vi "Shut down.vi"(8 "Error In":errorcluster, 11 "GUI":T1) -> ()   [LabVIEW 2011]
uses:
  Controls/Top Level Control.ctl
  <vilib>/NI/AMC/Message Queue.ctl
  <vilib>/NI/AMC/Message.ctl
  <vilib>/NI/Tools/Keyed Array/KeyedArray.ctl
  Controls/ListBox Test Record.ctl
  Controls/DVR of CSV Tests Data.ctl
  Controls/CSVs Tests Data.ctl
  Controls/Test Column Data.ctl
  Controls/Options DVR.ctl
  Controls/Options.ctl
  <userlib>/_MGI/Application Control/MGI Save & Restore Settings/MGI SRS Command Enum.ctl
  <vilib>/NI/AMC/AMC.lvlib
  <vilib>/NI/Tools/Keyed Array/Tools_KeyedArray.lvlib
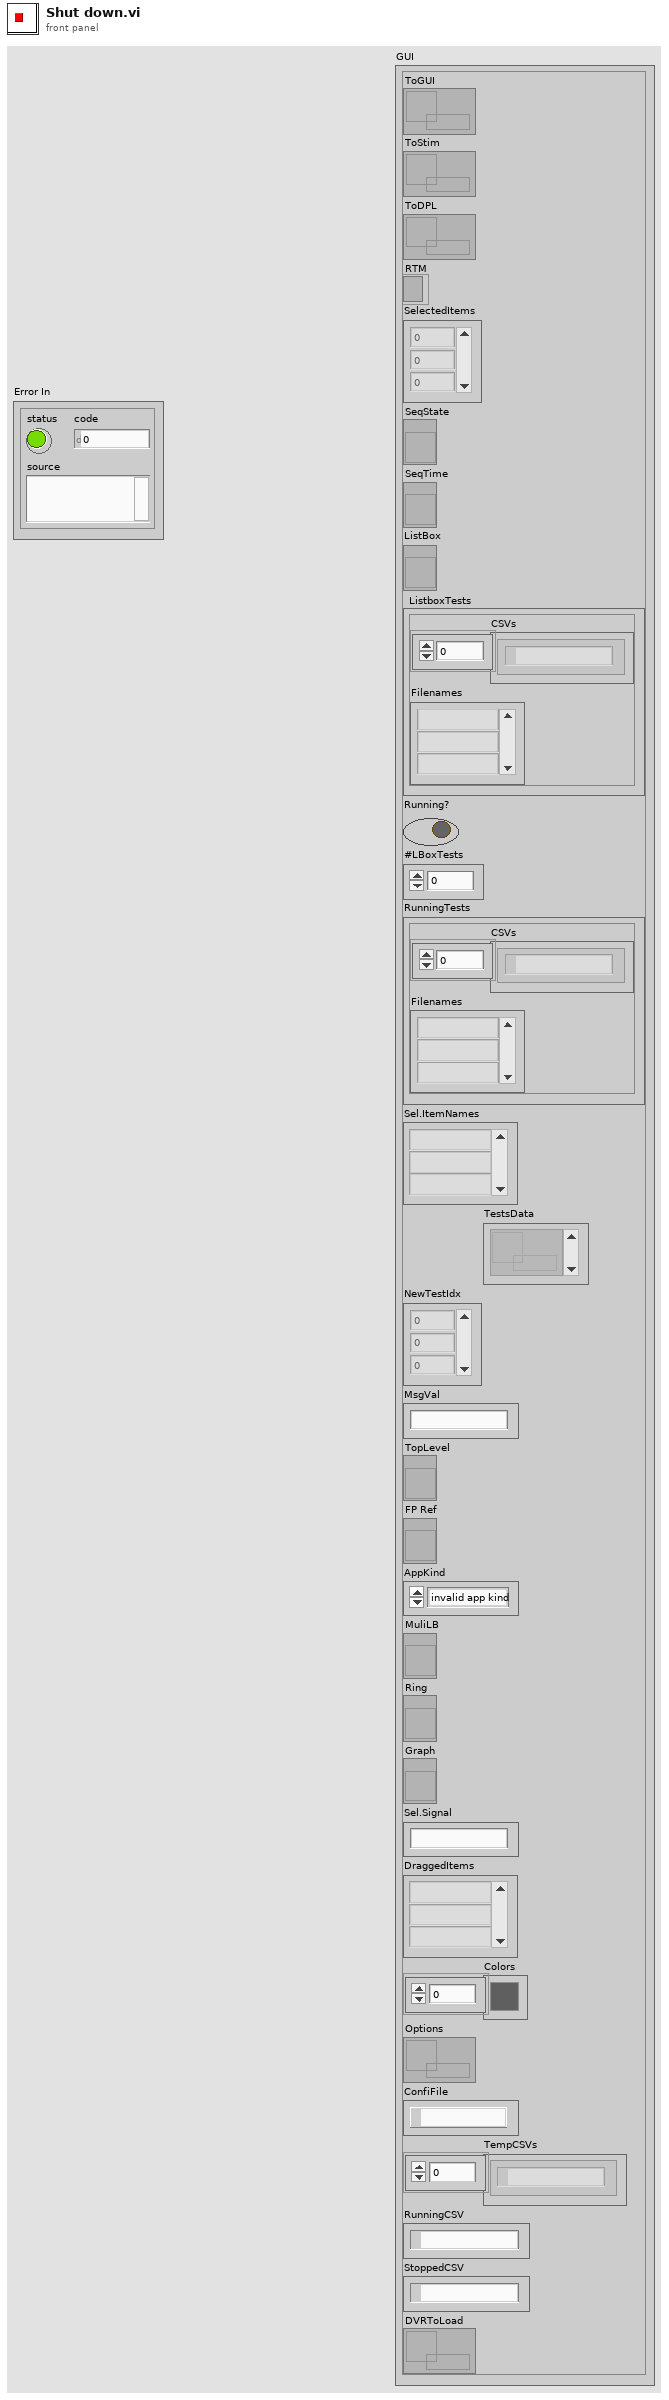
[diagram p1: front panel]
types:
  T1 = typedef "Top Level Control.ctl" = cluster{"ToGUI":T2, "ToStim":T2, "ToDPL":T2, "RTM":refnum<k9>, "SelectedItems":i32[], "SeqState":refnum<vi>, "SeqTime":refnum<vi>, "ListBox":refnum<vi>, "ListboxTests":T3, "Running?":bool, "#LBoxTests":i32, "RunningTests":T3, "Sel.ItemNames":string[], "TestsData":T4[], "NewTestIdx":i32[], "MsgVal":string, "TopLevel":refnum<vi>, "FP Ref":refnum<vi>, "AppKind":enum32{"invalid app kind", "Development System", "Run Time System", "Student Edition", "Embedded LabVIEW", "Evaluation", "Custom"}, "MuliLB":refnum<vi>, "Ring":refnum<vi>, "Graph":refnum<vi>, "Sel.Signal":string, "DraggedItems":string[], "Colors":u32[], "Options":T5, "ConfiFile":path, "TempCSVs":path[], "RunningCSV":path, "StoppedCSV":path, "DVRToLoad":T4}
  T2 = typedef "AMC.lvlib/Message Queue.ctl" = refnum<queue>
  T3 = typedef "ListBox Test Record.ctl" = cluster{"CSVs":path[], "Filenames":string[]}
  T4 = typedef "DVR of CSV Tests Data.ctl" = refnum<data-value>
  T5 = typedef "Options DVR.ctl" = refnum<data-value>
  T6 = typedef "MGI SRS Command Enum.ctl" = enum16{"Restore", "Save"}
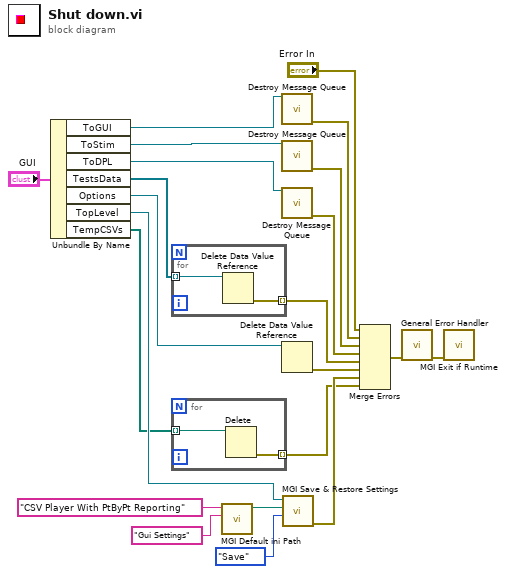
[diagram p0: block diagram]
diagram:
  n1 = Unbundle By Name("GUI") -> ("ToGUI"=w21:T2, "ToStim"=w20:T2, "ToDPL"=w19:T2, "TestsData"=w14:T4[], "Options"=w11:T5, "TopLevel"=w6:refnum<vi>, "TempCSVs"=w2:path[])
  n2 = for {
    tunnel: w14 -> [w24] mode=indexing
    tunnel: [w23] -> w13 mode=indexing
    n3 = Delete Data Value Reference(data value reference=w24) -> (error out=w23:errorcluster)  [unwired: 1 in, 1 out]
  }
  n4 = for {
    tunnel: w2 -> [w26] mode=indexing
    tunnel: [w25] -> w1 mode=indexing
    n5 = Delete(path (use dialog)=w26) -> (error out=w25:errorcluster)  [unwired: 4 in, 2 out]
  }
  n6 = call <userlib>:"MGI Default ini Path.vi"("File Name (Caller's Prefix)"="Gui Settings", "Folder Name (Caller's Prefix)"="CSV Player With PtByPt Reporting") -> ("Path"=w3:path)  [unwired: 9 in]
  n7 = call <vilib>:"Destroy Message Queue.vi"("message queue in"=w21) -> ("error out"=w17:errorcluster)  [unwired: 12 in, 2 out]
  n8 = call <vilib>:"Destroy Message Queue.vi"("message queue in"=w20) -> ("error out"=w16:errorcluster)  [unwired: 12 in, 2 out]
  n9 = call <vilib>:"Destroy Message Queue.vi"("message queue in"=w19) -> ("error out"=w15:errorcluster)  [unwired: 12 in, 2 out]
  n10 = Delete Data Value Reference(data value reference=w11) -> (error out=w10:errorcluster)  [unwired: 1 in, 1 out]
  n11 = call <userlib>:"MGI Save & Restore Settings.vi"("Command (Restore)"=MGI_SRS_Command_Enum."Save", "Path"=w3, "VI Reference In (Caller)"=w6) -> ("Error Out"=w7:errorcluster)  [unwired: 7 in, 1 out]
  n12 = Merge Errors("Error In", w17, w16, w15, w13, w10, w7, w1) -> (w12:errorcluster)
  n13 = call <vilib>:"General Error Handler.vi"("error in (no error)"=w12) -> ("error out"=w9:errorcluster)  [unwired: 10 in, 4 out]
  n14 = call <userlib>:"MGI Exit if Runtime.vi"("Error In (Dependency Only)"=w9) -> ()  [unwired: 11 in]
